vi "dispense_initial_HCl.vi"(0 "Dosimat In":T1={"Dosimat Port in"="COM1", "Error in"={"status"=FALSE, "code"=0, "source"=""}}, 5 "relay session in":T3={"VISA resource out"="COM12", "error out"={"status"=FALSE, "code"=0, "source"=""}}, 7 "Target EMF":dbl=0.001 min=0.001 max=2.5 format="%.2f", 9 "Initial HCl Increment":dbl=0.001 min=0.001 format="%.2f", 12 "Small Increment Size":dbl=0.001 min=0.001 max=2.5 format="%.2f", 13 "Probe to Follow":bool) -> (4 "Dosimat Out":T2={"Dosimat Port out"="COM1", "Error out"={"status"=FALSE, "code"=0, "source"=""}}, 6 "relay session out":T3={"VISA resource out"="COM12", "error out"={"status"=FALSE, "code"=0, "source"=""}})   [LabVIEW 2010]
panel:
  # "True for voltage 2, false for voltage 1"
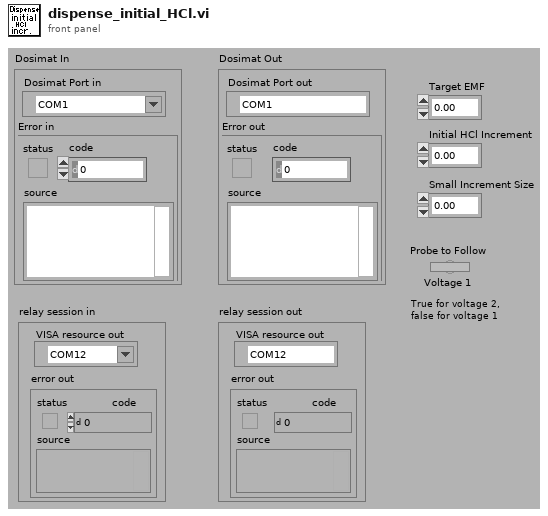
[diagram p1: front panel]
types:
  T1 = cluster{"Dosimat Port in":refnum<visa-resource-name>, "Error in":errorcluster}
  T2 = cluster{"Dosimat Port out":refnum<visa-resource-name>, "Error out":errorcluster}
  T3 = cluster{"VISA resource out":refnum<visa-resource-name>, "error out":errorcluster}
  T4 = cluster{"Dosimat Port Out":refnum<visa-resource-name>, "error out":errorcluster}
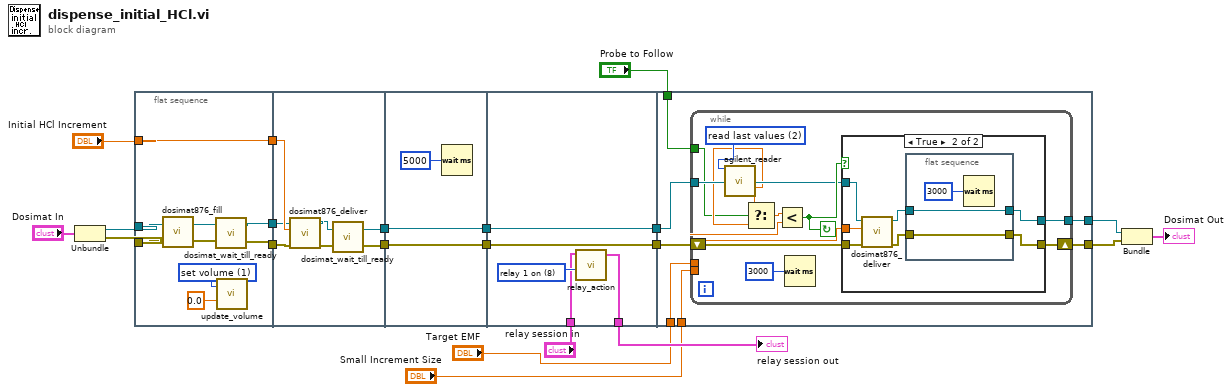
[diagram p0: block diagram]
diagram:
  n1 = Unbundle("Dosimat In") -> ("Dosimat Port in"=w6:refnum<visa-resource-name>, "Error in"=w5:errorcluster)
  n2 = flat-sequence {
    tunnel: "Initial HCl Increment" -> [w30]
    tunnel: [w30] -> w20
    tunnel: w6 -> [w29]
    tunnel: [w25] -> w19
    tunnel: w5 -> [w28]
    tunnel: [w24] -> w18
    tunnel: w20 -> [w37]
    tunnel: w19 -> [w36]
    tunnel: [w32] -> w17
    tunnel: w18 -> [w33]
    tunnel: [w31] -> w16
    tunnel: w17 -> [w39]
    tunnel: [w39] -> w15
    tunnel: w16 -> [w38]
    tunnel: [w38] -> w14
    tunnel: w15 -> [w45]
    tunnel: [w45] -> w13
    tunnel: w14 -> [w44]
    tunnel: [w44] -> w12
    tunnel: "relay session in" -> [w42]
    tunnel: [w41] -> w11
    tunnel: w13 -> [w52]
    tunnel: w12 -> [w51]
    tunnel: [w50] -> w4
    tunnel: [w49] -> w3
    tunnel: "Target EMF" -> [w48]
    tunnel: "Small Increment Size" -> [w47]
    tunnel: "Probe to Follow" -> [w46]
    frame #0 {
      w23 = u8 1 items=["add to volume", "set volume "] ("Action")
      n3 = call "dosimat876_fill.vi"("error in"=w28, "Dosimat Port In"=w29) -> ("error out"=w27:errorcluster, "Dosimat Port Out"=w26:refnum<visa-resource-name>)
      n4 = call "dosimat_wait_till_ready.vi"("error in"=w27, "Dosimat Port In"=w26) -> ("error out"=w24:errorcluster, "Dosimat Port Out"=w25:refnum<visa-resource-name>)
      n5 = call "update_volume.vi"("Volume In"=0.0, "Action"=w23) -> ()  [unwired: 1 out]
    }
    frame #1 {
      n6 = call "dosimat876_deliver.vi"("error in"=w33, "Volume"=w37, "Dosimat Port In"=w36) -> ("error out"=w34:errorcluster, "Dosimat Port Out"=w35:refnum<visa-resource-name>)  [unwired: 1 in, 2 out]
      n7 = call "dosimat_wait_till_ready.vi"("error in"=w34, "Dosimat Port In"=w35) -> ("error out"=w31:errorcluster, "Dosimat Port Out"=w32:refnum<visa-resource-name>)
    }
    frame #2 {
      n8 = Wait (ms)(milliseconds to wait=u32 5000) -> ()  [unwired: 1 out]
    }
    frame #3 {
      w43 = u8 8 items=["relay 1 on"=8, "relay 2 on"=9, "relay 3 on"=10, "relay 4 on"=11, "relay 1 off"=0, "relay 2 off"=1, "relay 3 off"=2, "relay 4 off"=3, "OpenAll"=30, "CloseAll"=29] ("Action 2")
      n9 = call "relay_action.vi"("relay session in"=w42, "Action"=w43) -> ("relay session out"=w41:T3)  [unwired: 6 in]
    }
    frame #4 {
      n10 = while {
        tunnel: w48 -> [w63]
        tunnel: w52 -> [w57]
        tunnel: [w60] -> w50
        shift-right: [w59] -> w49
        shift-left: w51 -> [w61]
        tunnel: w47 -> [w58]
        tunnel: w46 -> [w53]
        stop <- w64 continue-if-true
        w62 = u8 2 items=["read new values"=1, "read last values "=2] ("Action")
        n11 = call "agilent_reader.vi"("Action"=w62) -> ("Voltage 1"=w55:dbl, "Voltage 2"=w54:dbl)  [unwired: 3 in, 10 out]
        n12 = Select(t=w54, s=w53, f=w55) -> (s? t:f=w56:dbl)
        n13 = Less?(x=w56, y=w63) -> (x < y?=w64:bool)
        n14 = Wait (ms)(milliseconds to wait=3000) -> ()  [unwired: 1 out]
        n15 = case shown="True" w64 {
          tunnel: w58 -> [_ w73]
          tunnel: w57 -> [w66 w74]
          tunnel: w61 -> [w67 w72]
          tunnel: [w66 w69] -> w60
          tunnel: [w67 w68] -> w59
          frame False {
          }
          frame True {
            n16 = call "dosimat876_deliver.vi"("error in"=w72, "Volume"=w73, "Dosimat Port In"=w74) -> ("error out"=w70:errorcluster, "Dosimat Port Out"=w71:refnum<visa-resource-name>)  [unwired: 1 in, 2 out]
            n17 = flat-sequence {
              tunnel: [w76] -> w69
              tunnel: [w75] -> w68
              tunnel: w71 -> [w76]
              tunnel: w70 -> [w75]
              frame #0 {
                n18 = Wait (ms)(milliseconds to wait=3000) -> ()  [unwired: 1 out]
              }
            }
          }
        }
      }
    }
  }
  n19 = Bundle("Dosimat Port Out"=w4, "error out"=w3) -> (→"Dosimat Out":T4)  [unwired: 1 in]
  "relay session out" <- w11
